vi "Check_Messages.vi"(8 "Status/Errors in":refnum<vi>, 10 "Queues":T2) -> (0 "Status/Errors out":refnum<vi>, 1 "# Comparator data":i32, 2 "# One Second":i32, 3 "# errors":i32, 4 "Get/process":T1, 5 "# measurement data":i32)   [LabVIEW 2013]
uses:
  Controls/Queues.ctl
  Controls/One_Second.ctl
  Controls/GPS_Timestamp.ctl
  Controls/Command_Process_Messages.ctl
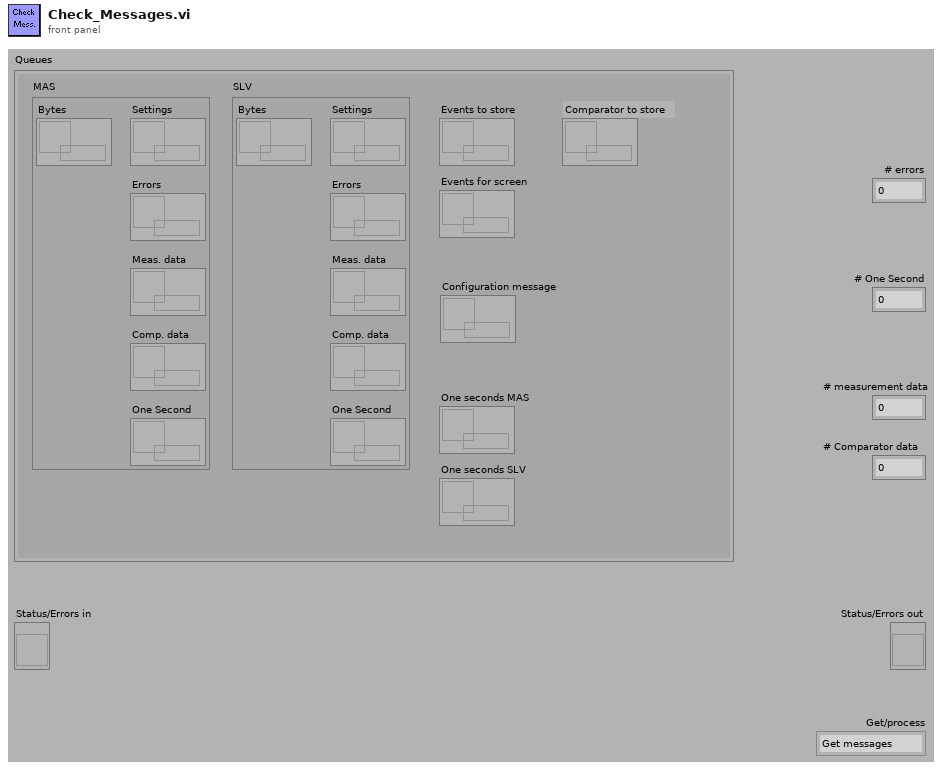
[diagram p1: front panel]
types:
  T1 = typedef "Command_Process_Messages.ctl" = enum16{"Get messages", "Process messages", "Stop loop", "No action"}
  T2 = typedef "Queues.ctl" = cluster{"MAS":cluster{"Bytes":refnum<queue>, "Settings":refnum<queue>, "Errors":refnum<queue>, "Meas. data":refnum<queue>, "One Second":refnum<queue>, "Comp. data":refnum<queue>}, "SLV":cluster{"Bytes":refnum<queue>, "Settings":refnum<queue>, "Errors":refnum<queue>, "Meas. data":refnum<queue>, "One Second":refnum<queue>, "Comp. data":refnum<queue>}, "Events to store":refnum<queue>, "Events for screen":refnum<queue>, "One seconds MAS":refnum<queue>, "One seconds SLV":refnum<queue>, "Configuration message":refnum<queue>, "Comparator to store":refnum<queue>}
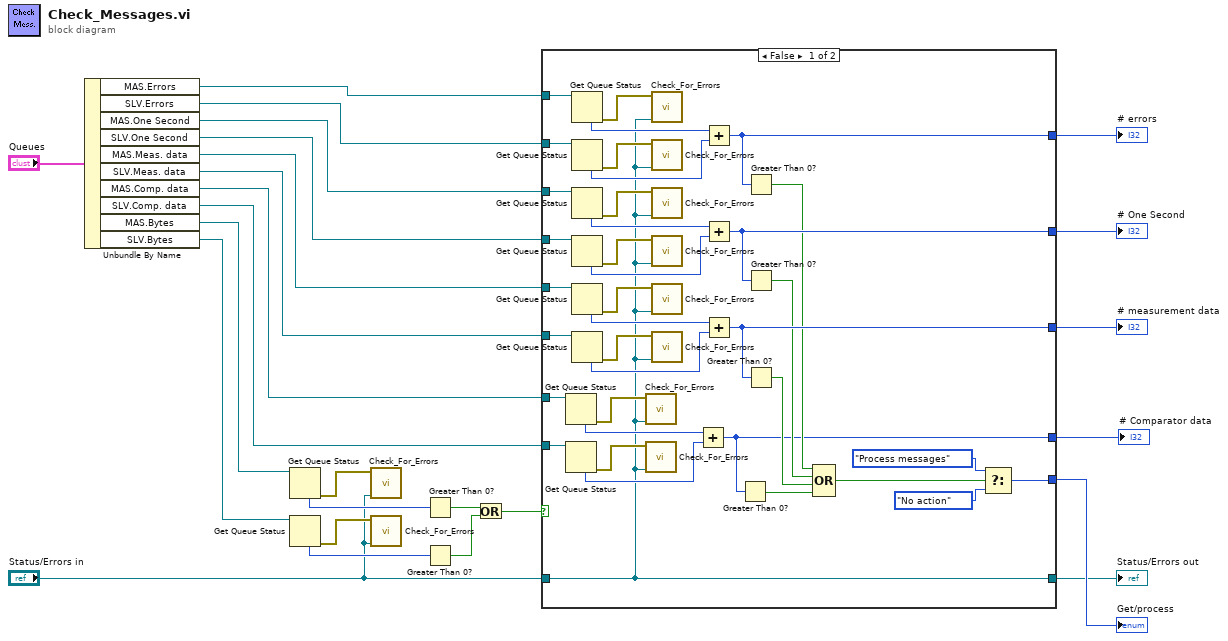
[diagram p0: block diagram]
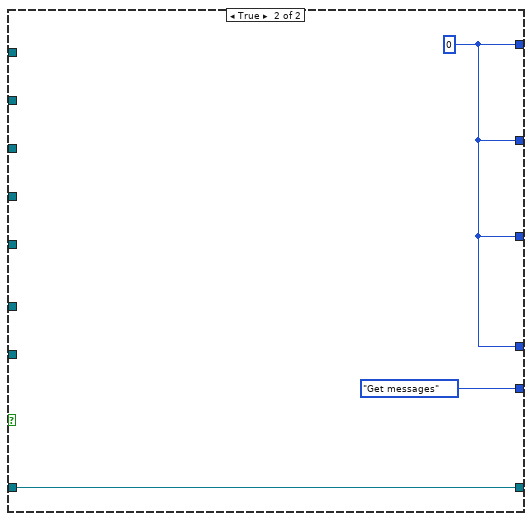
[diagram p2: hidden frame]
diagram:
  n1 = Unbundle By Name("Queues") -> ("MAS.Errors"=w23:refnum<queue>, "SLV.Errors"=w25:refnum<queue>, "MAS.One Second"=w24:refnum<queue>, "SLV.One Second"=w22:refnum<queue>, "MAS.Meas. data"=w21:refnum<queue>, "SLV.Meas. data"=w20:refnum<queue>, "MAS.Comp. data"=w5:refnum<queue>, "SLV.Comp. data"=w4:refnum<queue>, "MAS.Bytes"=w6:refnum<queue>, "SLV.Bytes"=w7:refnum<queue>)
  n2 = Get Queue Status(queue=w6) -> (error out=w19:errorcluster, # elements in queue=w11:i32)  [unwired: 1 in, 7 out]
  n3 = Get Queue Status(queue=w7) -> (error out=w18:errorcluster, # elements in queue=w10:i32)  [unwired: 1 in, 7 out]
  n4 = call "Check_For_Errors.vi"("Status/Errors in"="Status/Errors in", "error in"=w19) -> ()  [unwired: 10 out]
  n5 = call "Check_For_Errors.vi"("Status/Errors in"="Status/Errors in", "error in"=w18) -> ()  [unwired: 10 out]
  n6 = Greater Than 0?(x=w11) -> (x > 0?=w9:bool)
  n7 = Greater Than 0?(x=w10) -> (x > 0?=w8:bool)
  n8 = Or(x=w9, y=w8) -> (x .or. y?=w13:bool)
  n9 = case shown="False" w13 {
    tunnel: w25 -> [w62 _]
    tunnel: w24 -> [w61 _]
    tunnel: w23 -> [w60 _]
    tunnel: w22 -> [w59 _]
    tunnel: w21 -> [w58 _]
    tunnel: w20 -> [w57 _]
    tunnel: [w43 w64] -> w16
    tunnel: [w42 w64] -> w15
    tunnel: [w44 w64] -> w14
    tunnel: "Status/Errors in" -> [w26 w63]
    tunnel: [w39 Command_Process_Messages."Get messages" ("Get/process")] -> w12
    tunnel: w5 -> [w31 _]
    tunnel: w4 -> [w30 _]
    tunnel: [w28 w64] -> w3
    tunnel: [w26 w63] -> w1
    frame False {
      n10 = Get Queue Status(queue=w31) -> (error out=w35:errorcluster, # elements in queue=w32:i32)  [unwired: 1 in, 7 out]
      n11 = Get Queue Status(queue=w30) -> (error out=w34:errorcluster, # elements in queue=w33:i32)  [unwired: 1 in, 7 out]
      n12 = Get Queue Status(queue=w60) -> (error out=w56:errorcluster, # elements in queue=w50:i32)  [unwired: 1 in, 7 out]
      n13 = Get Queue Status(queue=w62) -> (error out=w55:errorcluster, # elements in queue=w49:i32)  [unwired: 1 in, 7 out]
      n14 = Get Queue Status(queue=w61) -> (error out=w54:errorcluster, # elements in queue=w48:i32)  [unwired: 1 in, 7 out]
      n15 = Get Queue Status(queue=w59) -> (error out=w53:errorcluster, # elements in queue=w47:i32)  [unwired: 1 in, 7 out]
      n16 = Get Queue Status(queue=w58) -> (error out=w52:errorcluster, # elements in queue=w36:i32)  [unwired: 1 in, 7 out]
      n17 = Get Queue Status(queue=w57) -> (error out=w51:errorcluster, # elements in queue=w38:i32)  [unwired: 1 in, 7 out]
      n18 = call "Check_For_Errors.vi"("Status/Errors in"=w26, "error in"=w35) -> ()  [unwired: 10 out]
      n19 = call "Check_For_Errors.vi"("Status/Errors in"=w26, "error in"=w34) -> ()  [unwired: 10 out]
      n20 = call "Check_For_Errors.vi"("Status/Errors in"=w26, "error in"=w56) -> ()  [unwired: 10 out]
      n21 = call "Check_For_Errors.vi"("Status/Errors in"=w26, "error in"=w55) -> ()  [unwired: 10 out]
      n22 = call "Check_For_Errors.vi"("Status/Errors in"=w26, "error in"=w54) -> ()  [unwired: 10 out]
      n23 = call "Check_For_Errors.vi"("Status/Errors in"=w26, "error in"=w53) -> ()  [unwired: 10 out]
      n24 = call "Check_For_Errors.vi"("Status/Errors in"=w26, "error in"=w52) -> ()  [unwired: 10 out]
      n25 = call "Check_For_Errors.vi"("Status/Errors in"=w26, "error in"=w51) -> ()  [unwired: 10 out]
      n26 = Add(x=w32, y=w33) -> (x+y=w28:i32)
      n27 = Add(x=w50, y=w49) -> (x+y=w42:i32)
      n28 = Add(x=w48, y=w47) -> (x+y=w43:i32)
      n29 = Add(x=w36, y=w38) -> (x+y=w44:i32)
      n30 = Greater Than 0?(x=w28) -> (x > 0?=w29:bool)
      n31 = Greater Than 0?(x=w42) -> (x > 0?=w41:bool)
      n32 = Greater Than 0?(x=w43) -> (x > 0?=w40:bool)
      n33 = Greater Than 0?(x=w44) -> (x > 0?=w37:bool)
      n34 = Compound Arithmetic op=OR(w41, w40, w37, w29) -> (w27:bool)
      n35 = Select(t=Command_Process_Messages."Process messages" ("Get/process"), s=w27, f=Command_Process_Messages."No action" ("Get/process")) -> (s? t:f=w39:T1)
    }
    frame True {
      w64 = 0
    }
  }
  "# One Second" <- w16
  "# errors" <- w15
  "# measurement data" <- w14
  "Get/process" <- w12
  "Status/Errors out" <- w1
  "# Comparator data" <- w3
